vi "provide_OME_component_parameters.vi"(7 "cluster name":string, 8 "error in (no error)":errorcluster, 9 "cluster variant":variant, 10 "XMLElement in":refnum<class "XMLElement.lvclass">) -> (0 "error out":errorcluster, 2 "XMLElement out":refnum<class "XMLElement.lvclass">)   [LabVIEW 2010, in "GenericComponent.lvclass"]
uses:
  GenericComponent.lvclass
  XMLElement/XMLElement/XMLElement.lvclass
  SoftwareParameter/SoftwareParameter/SoftwareParameter.lvclass
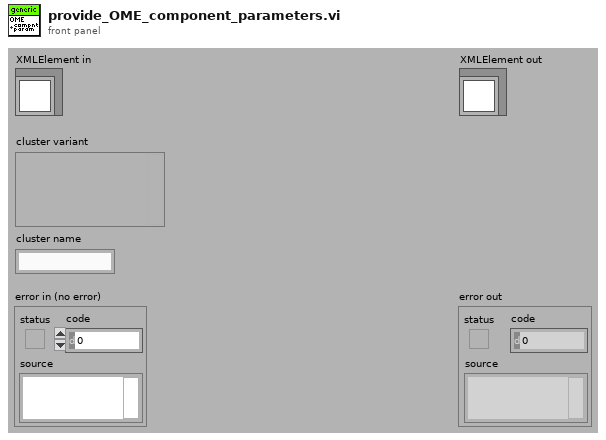
[diagram p1: front panel]
types:
  T1 = typedef "Type Descriptor Enumeration__ogtk.ctl" = enum8{"<Null>", "I8", "I16", "I32", "I64", "U8", "U16", "U32", "U64", "SGL", "DBL", "EXT", "CSG", "CDB", "CXT", "0x0F", "0x10", "0x11", "0x12", "0x13", "0x14", "Enum U8", "Enum U16", "Enum U32", "Enum U64", "SGL PQ", "DBL PQ", "EXT PQ", "CSG PQ", "CDB PQ", "CXT PQ", "0x1F", "0x20", "Boolean", "0x22", "0x23", "0x24", "0x25", "0x26", "0x27", "0x28", "0x29", "0x2A", "0x2B", "0x2C", "0x2D", "0x2E", "0x2F", "String", "0x31", "Path", "Pict", "0x34", "0x35", "0x36", "DAQ", "0x38", "0x39", "0x3A", "0x3B", "0x3C", "0x3D", "0x3E", "0x3F", "Array", "0x41", "0x42", "0x43", "0x44", "0x45", "0x46", "0x47", "0x48", "0x49", "0x4A", "0x4B", "0x4C", "0x4D", "0x4E", "0x4F", "Cluster", "0x51", "0x52", "Variant", "Waveform", "0x55", "0x56", "0x57", "0x58", "0x59", "0x5A", "0x5B", "0x5C", "0x5D", "0x5E", "0x5F", "0x60", "0x61", "0x62", "0x63", "0x64", "0x65", "0x66", "0x67", "0x68", "0x69", "0x6A", "0x6B", "0x6C", "0x6D", "0x6E", "0x6F", "Refnum"}
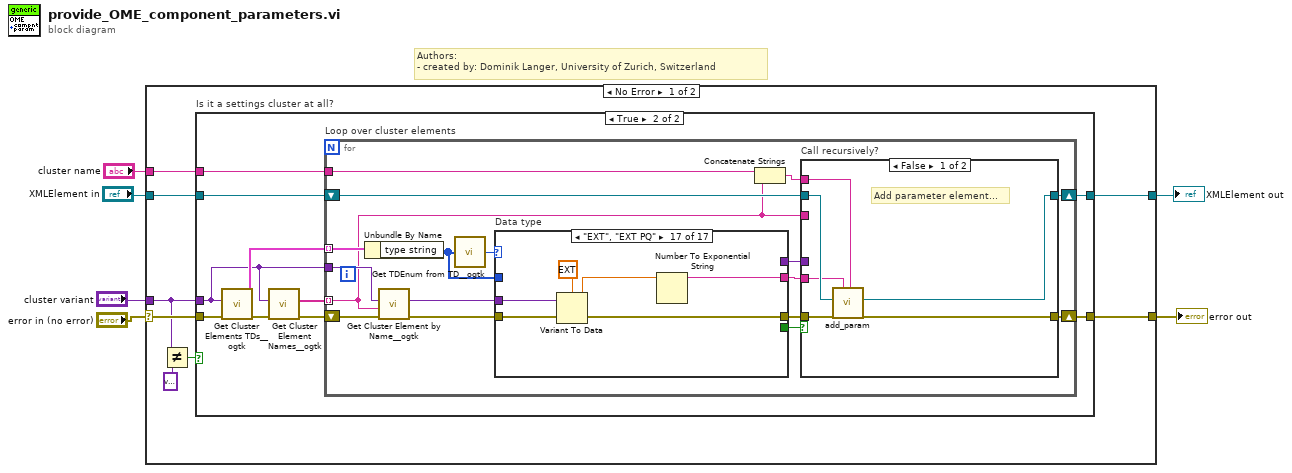
[diagram p0: block diagram]
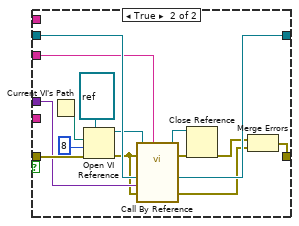
[diagram p3: hidden frame]
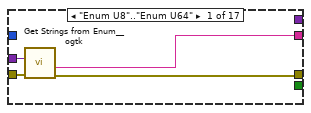
[diagram p4: hidden frame]
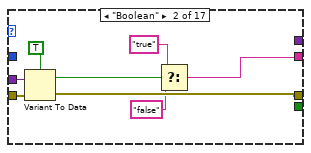
[diagram p5: hidden frame]
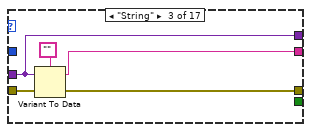
[diagram p6: hidden frame]
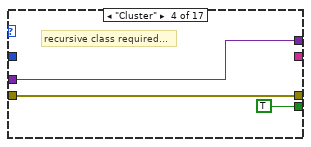
[diagram p7: hidden frame]
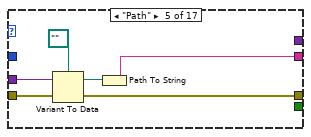
[diagram p8: hidden frame]
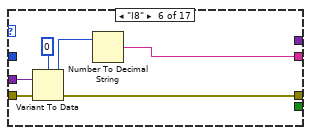
[diagram p9: hidden frame]
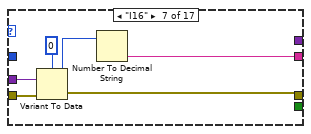
[diagram p10: hidden frame]
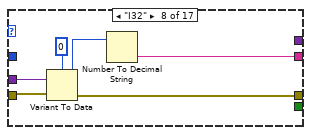
[diagram p11: hidden frame]
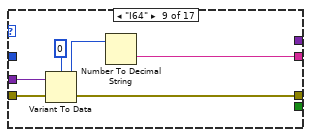
[diagram p12: hidden frame]
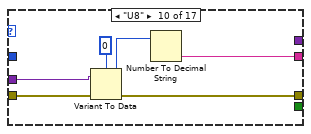
[diagram p13: hidden frame]
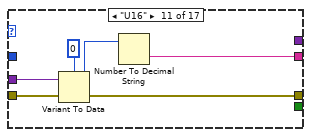
[diagram p14: hidden frame]
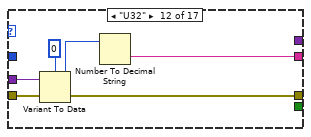
[diagram p15: hidden frame]
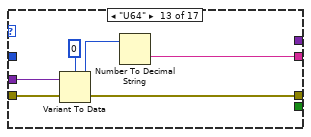
[diagram p16: hidden frame]
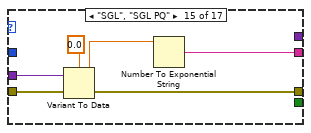
[diagram p18: hidden frame]
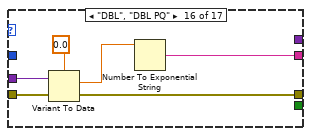
[diagram p19: hidden frame]
diagram:
  # "Authors: \n- created by: Dominik Langer, University of Zurich, Switzerland"
  n1 = case shown="No Error" "error in (no error)" {
    selector: "error in (no error)" -> [w14 w159]
    tunnel: [w13 w159] -> w5
    tunnel: "cluster variant" -> [w10 _]
    tunnel: "XMLElement in" -> [w12 w158]
    tunnel: [w11 w158] -> w2
    tunnel: "cluster name" -> [w7 _]
    frame No Error {
      n2 = Not Equal?(x=w10, y=variant ("variant")) -> (x != y?=w8:bool)
      n3 = case "Is it a settings cluster at all?" shown="True" w8 {
        tunnel: w14 -> [w16 w26]
        tunnel: [w16 w24] -> w13
        tunnel: w12 -> [w15 w23]
        tunnel: [w15 w22] -> w11
        tunnel: w10 -> [_ w18]
        tunnel: w7 -> [_ w17]
        frame False {
        }
        frame True {
          n4 = call <userlib>:"Get Cluster Elements TDs__ogtk.vi"("error in (no error)"=w26, "Cluster"=w18) -> ("error out"=w25:errorcluster, "type strings"=w21:cluster{"type string":i16[]}[])  [unwired: 8 in]
          n5 = call <userlib>:"Get Cluster Element Names__ogtk.vi"("error in (no error)"=w25, "Cluster"=w18) -> ("error out"=w20:errorcluster, "Element Names"=w19:string[])  [unwired: 8 in]
          n6 = for "Loop over cluster elements" {
            tunnel: w19 -> [w28] mode=indexing
            shift-right: [w30] -> w24
            shift-left: w20 -> [w35]
            tunnel: w18 -> [w43]
            tunnel: w21 -> [w42] mode=indexing
            shift-right: [w37] -> w22
            shift-left: w23 -> [w38]
            tunnel: w17 -> [w29]
            n7 = Unbundle By Name(w42) -> ("type string"=w33:i16[])
            n8 = call <userlib>:"Get Cluster Element by Name__ogtk.vi"("error in (no error)"=w35, "Element Name"=w28, "Cluster"=w43) -> ("error out"=w34:errorcluster, "VElement"=w41:variant)  [unwired: 6 in, 1 out]
            n9 = call <userlib>:"Get TDEnum from TD__ogtk.vi"("Type Descriptor"=w33) -> ("Type Descriptor Enumeration"=w31:T1)  [unwired: 4 in]
            n10 = case "Data type" shown="\"EXT\", \"EXT PQ\"" w31 {
              tunnel: w34 -> [w68 w75 w81 w84 w89 w95 w100 w104 w112 w118 w122 w130 w134 w139 w143 w150 w156]
              tunnel: w41 -> [w67 w76 w77 w82 w88 w96 w99 w103 w111 w116 w121 w129 w133 _ w144 w149 w154]
              tunnel: [w66 w69 w78 _ w85 w92 w97 w106 w109 w115 w124 w127 w136 _ w140 w146 w152] -> w36
              tunnel: [w65 w71 w79 w84 w87 w91 w98 w105 w110 w117 w123 w128 w135 w139 w142 w148 w155] -> w40
              tunnel: [_ _ _ TRUE _ _ _ _ _ _ _ _ _ _ _ _ _] -> w32
              tunnel: [_ _ w77 w82 _ _ _ _ _ _ _ _ _ _ _ _ _] -> w39
              tunnel: w33 -> [_ _ _ _ _ _ _ _ _ _ _ _ _ _ _ _ _]
              frame "Enum U8".."Enum U64" {
                n11 = call <userlib>:"Get Strings from Enum__ogtk.vi"("error in (no error)"=w68, "Enum"=w67) -> ("error out"=w65:errorcluster, "String Value"=w66:string)  [unwired: 6 in, 2 out]
              }
              frame "Boolean" {
                n12 = Variant To Data(error in=w75, Variant=w76, type=TRUE) -> (error out=w71:errorcluster, data=w73:bool)
                n13 = Select(t="true", s=w73, f="false") -> (s? t:f=w69:string)
              }
              frame "String" {
                n14 = Variant To Data(error in=w81, Variant=w77, type="") -> (error out=w79:errorcluster, data=w78:string)
              }
              frame "Cluster" {
                # "recursive class required..."
              }
              frame "Path" {
                n15 = Variant To Data(error in=w89, Variant=w88, type=path "") -> (error out=w87:errorcluster, data=w86:path)
                n16 = Path To String(path=w86) -> (string=w85:string)
              }
              frame "I8" {
                n17 = Variant To Data(error in=w95, Variant=w96, type=i8 0) -> (error out=w91:errorcluster, data=w93:i8)
                n18 = Number To Decimal String(number=w93) -> (decimal integer string=w92:string)  [unwired: 1 in]
              }
              frame "I16" {
                n19 = Variant To Data(error in=w100, Variant=w99, type=i16 0) -> (error out=w98:errorcluster, data=w101:i16)
                n20 = Number To Decimal String(number=w101) -> (decimal integer string=w97:string)  [unwired: 1 in]
              }
              frame "I32" {
                n21 = Variant To Data(error in=w104, Variant=w103, type=0) -> (error out=w105:errorcluster, data=w107:i32)
                n22 = Number To Decimal String(number=w107) -> (decimal integer string=w106:string)  [unwired: 1 in]
              }
              frame "I64" {
                n23 = Variant To Data(error in=w112, Variant=w111, type=i64 0) -> (error out=w110:errorcluster, data=w113:i64)
                n24 = Number To Decimal String(number=w113) -> (decimal integer string=w109:string)  [unwired: 1 in]
              }
              frame "U8" {
                n25 = Variant To Data(error in=w118, Variant=w116, type=u8 0) -> (error out=w117:errorcluster, data=w119:u8)
                n26 = Number To Decimal String(number=w119) -> (decimal integer string=w115:string)  [unwired: 1 in]
              }
              frame "U16" {
                n27 = Variant To Data(error in=w122, Variant=w121, type=u16 0) -> (error out=w123:errorcluster, data=w125:u16)
                n28 = Number To Decimal String(number=w125) -> (decimal integer string=w124:string)  [unwired: 1 in]
              }
              frame "U32" {
                n29 = Variant To Data(error in=w130, Variant=w129, type=u32 0) -> (error out=w128:errorcluster, data=w131:u32)
                n30 = Number To Decimal String(number=w131) -> (decimal integer string=w127:string)  [unwired: 1 in]
              }
              frame "U64" {
                n31 = Variant To Data(error in=w134, Variant=w133, type=u64 0) -> (error out=w135:errorcluster, data=w137:u64)
                n32 = Number To Decimal String(number=w137) -> (decimal integer string=w136:string)  [unwired: 1 in]
              }
              frame Default {
              }
              frame "SGL", "SGL PQ" {
                n33 = Variant To Data(error in=w143, Variant=w144, type=sgl 0.0) -> (error out=w142:errorcluster, data=w141:sgl)
                n34 = Number To Exponential String(number=w141) -> (E-format string=w140:string)  [unwired: 3 in]
              }
              frame "DBL", "DBL PQ" {
                n35 = Variant To Data(error in=w150, Variant=w149, type=0.0) -> (error out=w148:errorcluster, data=w147:dbl)
                n36 = Number To Exponential String(number=w147) -> (E-format string=w146:string)  [unwired: 3 in]
              }
              frame "EXT", "EXT PQ" {
                n37 = Variant To Data(error in=w156, Variant=w154, type=ext 0.0) -> (error out=w155:errorcluster, data=w153:ext)
                n38 = Number To Exponential String(number=w153) -> (E-format string=w152:string)  [unwired: 3 in]
              }
            }
            n39 = Concatenate Strings(w29, w28) -> (w27:string)
            n40 = case "Call recursively?" shown="False" w32 {
              tunnel: w40 -> [w49 w64]
              tunnel: [w48 w63] -> w30
              tunnel: w39 -> [_ w60]
              tunnel: w38 -> [w47 w62]
              tunnel: [w46 w61] -> w37
              tunnel: w36 -> [w45 _]
              tunnel: w28 -> [_ w50]
              tunnel: w27 -> [w44 _]
              frame False {
                # "Add parameter element..."
                n41 = call "add_param.vi"("name"=w44, "value"=w45, "error in (no error)"=w49, "parent element in"=w47) -> ("error out"=w48:errorcluster, "parent element out"=w46:refnum<class "XMLElement.lvclass">)  [unwired: 5 in, 1 out]
              }
              frame True {
                n42 = Current VI's Path() -> (path=w54:path)
                n43 = Open VI Reference(type specifier VI Refnum (for type only)=refnum<vi> refnum, vi path=w54, options=8, error in (no error)=w64) -> (vi reference=w58:refnum<vi>, error out=w56:errorcluster)  [unwired: 2 in]
                n44 = call-by-ref "?"(reference=w58, error in=w56, "cluster name"=w50, 8:"error in (no error)"=w56, "cluster variant"=w60, "XMLElement in"=w62) -> (reference out=w51:refnum<vi>, error out=w53:errorcluster, 0:"error out"=w59:errorcluster, "XMLElement out"=w61:refnum<class "XMLElement.lvclass">)  [unwired: 6 in]
                n45 = Close Reference(reference=w51, error in (no error)=w53) -> (error out=w52:errorcluster)
                n46 = Merge Errors(w52, w59) -> (w63:errorcluster)
              }
            }
          }
        }
      }
    }
    frame Error {
    }
  }
  "error out" <- w5
  "XMLElement out" <- w2
